vi "카운트(시프트레지스터).vi"() -> ()   [LabVIEW 2020]
panel:
  out "출력 배열":dbl[](array[numeric])
  out "추가된 배열":dbl[](array[numeric])
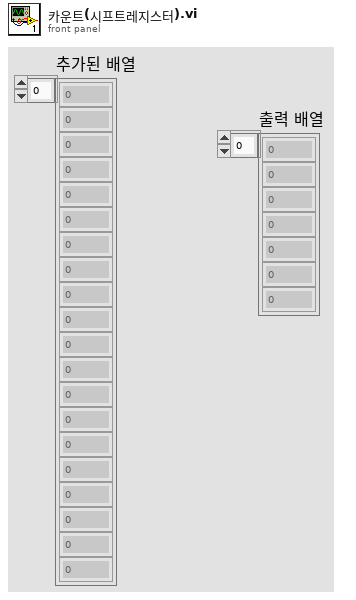
[diagram p1: front panel]
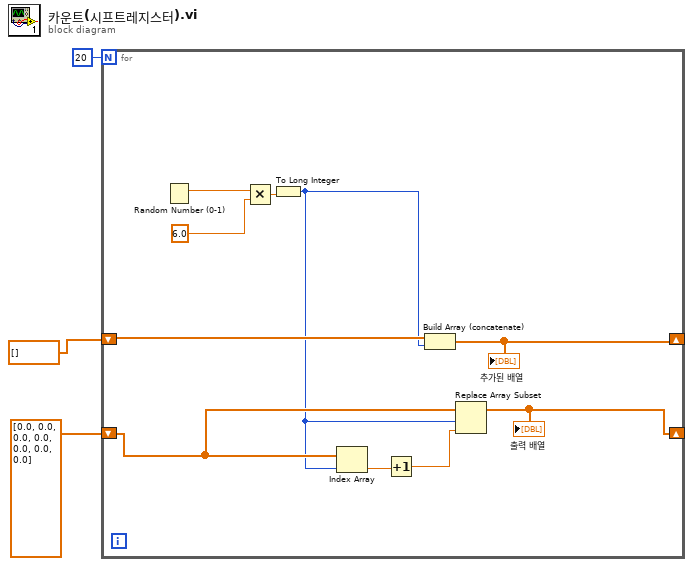
[diagram p0: block diagram]
diagram:
  n1 = for {
    N: 20 -> [_]
    shift-right: [w9] -> _
    shift-left: dbl[] [] -> [w10]
    shift-right: [w4] -> _
    shift-left: dbl[] [0.0, 0.0, 0.0, 0.0, 0.0, 0.0, 0.0] -> [w8]
    n2 = Random Number (0-1)() -> (number: 0 to 1=w13:dbl)
    n3 = Multiply(x=w13, y=6.0 ("x")) -> (x*y=w11:dbl)
    n4 = To Long Integer(number=w11) -> (32bit integer=w5:i32)
    n5 = Index Array(array=w8, index=w5) -> (element=w7:dbl)
    n6 = Increment(x=w7) -> (x+1=w6:dbl)
    n7 = Build Array (concatenate)(w10, w5) -> (w9:dbl[])
    "추가된 배열" <- w9
    n8 = Replace Array Subset(array=w8, new element=w6, index=w5) -> (w4:dbl[])
    "출력 배열" <- w4
  }
